vi "FPGA cRIOMain_v10.vi"() -> ()   [LabVIEW 2019]
doc: "Main FPGA VI\nUse the bitfile generated by this VI in the real-time code.\n\nv5: Use 16-pt MA filter in AI loop"
uses:
  TypeDefs/AO mode TabCtrl.ctl
  TypeDefs/SamplingModeEnum.ctl
  TypeDefs/AI_channelEnum.ctl
  <vilib>/Platform/TimedLoop/XDataNode/timing_clust.ctl
  <vilib>/Platform/TimedLoop/XDataNode/nitl_modes.ctl
  <vilib>/Platform/TimedLoop/XDataNode/wakeup.ctl
  <vilib>/rvi/Emulation/niFpgaGetClockAttributes.vi
  <vilib>/rvi/Emulation/niFpgaSctlEmulationGetInTimedLoop.vi
  <vilib>/rvi/Emulation/niFpgaEmulationReportErrorSimple.vi
  <vilib>/rvi/eio/common/nirviEmuTemplateMethod_errors.vi
  <vilib>/rvi/Emulation/niFpgaEmulationIsFPGAContextNoSignature.vi
  <vilib>/rvi/errors/niFpgaSetErrorForExecOnDevCompSimple.vi
  <vilib>/rvi/eio/common/nirviEmuReportErrorAndStop.vi
  <vilib>/rvi/DataTransferAndStorage/Container/Common/niFpgaContainerGetUniqueNameForEmu.vi
  <vilib>/rvi/FIFO/Fifo_Resource/nirvififoEmulationSetSize.vi
  <vilib>/rvi/FIFO/Fifo_Resource/nirviFifoEmulationQueueMgr.vi
  <instcachedir>/0/nirviFifoEmulationQueueMgr_E5CAEC123FF24DC58D834DCA3CDAA9B5.lvgen/nirviFifoEmulationQueueMgr_E5CAEC123FF24DC58D834DCA3CDAA9B5_000.vi
  <vilib>/rvi/FIFO/Fifo_Resource/nirvififoEmulationDetermineInputValidOut.vi
  <vilib>/rvi/FIFO/Fifo_Resource/nirvififoEmulationCreateLock.vi
  <vilib>/rvi/Emulation/niFpgaProcessEmulError.vi
  <vilib>/rvi/FIFO/Fifo_Resource/nirvififoEmulationObtainLock.vi
  <vilib>/rvi/FIFO/Fifo_Resource/nirvififoEmulationReleaseLock.vi
  <vilib>/rvi/occurrence/nirviWaitOnOccurrenceBase.vi
  <vilib>/rvi/errors/nirviReportUnexpectedCaseInternalError.vi
  <vilib>/rvi/errors/nirviReportUnexpectedCaseInternalError (U32).vi
  <vilib>/rvi/Emulation/niFpgaCriticalErrorInLSC.vi
  <instcachedir>/0/nirviFifoEmulationQueueMgr_E5CAEC123FF24DC58D834DCA3CDAA9B5.lvgen/nirviFifoEmulationQueueMgr_E5CAEC123FF24DC58D834DCA3CDAA9B5_006.vi
  <vilib>/Utility/error.llb/Clear Errors.vi
  <vilib>/rvi/Memory/Memory_Emulation/niFpgaMemoryEmulationCacheClearOnFirstRun.vi
  <vilib>/rvi/Memory/Memory_Emulation/nirvimemoryEmulationManagerCache_MakeExclusive.vi
  <vilib>/rvi/Memory/Memory_Emulation/niFpgaMemoryEmulationValidateCache.vi
  <vilib>/rvi/Memory/Memory_Emulation/nirvimemoryEmulationManagerCache_InsertValue.vi
  <vilib>/rvi/Memory/Memory_Emulation/nirvimemoryEmulationManagerCache_ReleaseExclusive.vi
  <vilib>/rvi/Memory/Memory_Emulation/nirvimemoryEmulationManagerCache_GetValue.vi
  <vilib>/rvi/Memory/Memory_Emulation/nirvimemoryEmulationManagerCache_SetValue.vi
  <vilib>/rvi/Analysis/common/codeGenErrors/XNode/niFpgaXNodeCodeGenErrorHandle.vi
  <vilib>/eio/EIONode/EIONode.xnode
  <vilib>/rvi/DataTransferAndStorage/Container/XNode/niFpgaContainer.xnode
  <vilib>/rvi/FIFO/Fifo_Resource/nirvififoEmulationWrite.vi
  <vilib>/rvi/FIFO/Fifo_Resource/nirvififoEmulationRead.vi
  <vilib>/rvi/DataTransferAndStorage/Register/Emulation/niFpgaRegisterEmulation.vi
  <vilib>/rvi/FXPMathLib/FxpMul/XNode/nifxpmath_Multiplier.xnode
  <vilib>/rvi/Analysis/measure/LMRsmpl/XNode/niFPGA Rational Resampler.xnode
  <vilib>/Platform/TimedLoop/XDataNode/XDataNode.xnode
  <vilib>/rvi/FXPMathLib/sim/FxpSim.dll
  <vilib>/Platform/TimedLoop/XDataNode/XDNodeRunTimeDep.lvlib
panel:
  out "AI M loop time [ticks]":u32
  out "FPGA AI DMA\nOverflow?":bool
  out "AI Processing\nLoop Rate to high?":bool
  in  "AI Process Time [ticks]":u32=125
  in  "Select Channel":T1
  out "Unable to\nsample at desired\nSample Rate?":bool
  out "Processing Loop time [ticks]":u32
  in  "Sampling Mode":T2
  in  "AO mode":T3
  in  "AO Out [V]":fxp<+/-,18,5> format="%#.6g"
  in  "AO enable?":bool
  out "AI In [V]":fxp<+/-,25,5> format="%#.6g"
  out "FPGA AO DMA\nOverflow?":bool
  out "Int. Output":fxp<+/-,20,5> format="%.17g"
  out "Raw AI Input":fxp<+/-,25,5> format="%.21g"
  in  "Sample Time [ticks]":u32=125
  out "AO Loop time [ticks]":u32
  out "AI Loop time [ticks]":u32
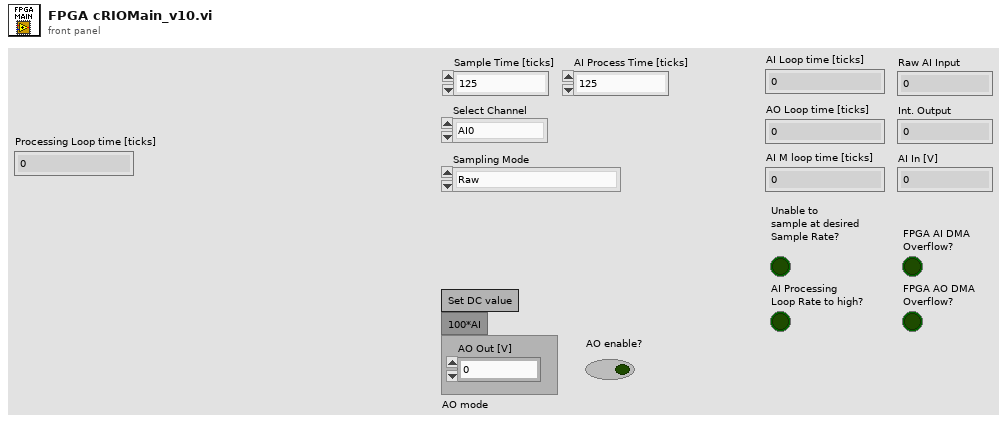
[diagram p1: front panel]
types:
  T1 = typedef "AI_channelEnum.ctl" = enum16{"AI0", "AI1", "AI2", "AI3"}
  T2 = typedef "SamplingModeEnum.ctl" = enum16{"Raw", "M64 (ReSpl)", "M128 (ReSpl)", "4pt MA (AI) + M64 (ReSpl)", "LPF (Proc.)", "4pt MA (AI) + LPF (Proc.)", "4pt MA (Proc.) + LPF (Proc.)"}
  T3 = typedef "AO mode TabCtrl.ctl" = enum32{"Set DC value", "100*AI"}
  T4 = typedef "XDNodeRunTimeDep.lvlib/timing_clust.ctl" = cluster{"Expected End [f-1]":u64, "Actual End [f-1]":u64, "Finished Late? [f-1]":bool, "Expected End [i-1]":u64, "Actual End [i-1]":u64, "Finished Late? [i-1]":bool, "Expected Start [i]":u64, "Actual Start [i]":u64, "Expected Start [f]":u64, "Actual Start [f]":u64, "Source Name":string, "Structure Name":string, "Period":i64, "Deadline":i64, "Offset":i64, "Start":i64, "Priority":i32, "Timeout":i32, "Mode":T5, "Wakeup Reason":T6, "Error":errorcluster, "Source Type":string, "Secondary Source Type":string, "Global End Time":u64, "Global Start Time":u64, "Frame Duration":u64, "Iteration Duration":u64, "Assigned CPU":i32, "I/O Scan Engine Mode":u32}
  T5 = typedef "XDNodeRunTimeDep.lvlib/nitl_modes.ctl" = enum32{"No Change", "Process missed periods, maintain original phase", "Discard missed periods, maintain original phase", "Process missed periods, ignore original phase", "Discard missed periods, ignore original phase"}
  T6 = typedef "XDNodeRunTimeDep.lvlib/wakeup.ctl" = enum32{"Normal", "Aborted", "Asynchronous wakeup", "Timing source error", "Timed loop error", "Timeout"}
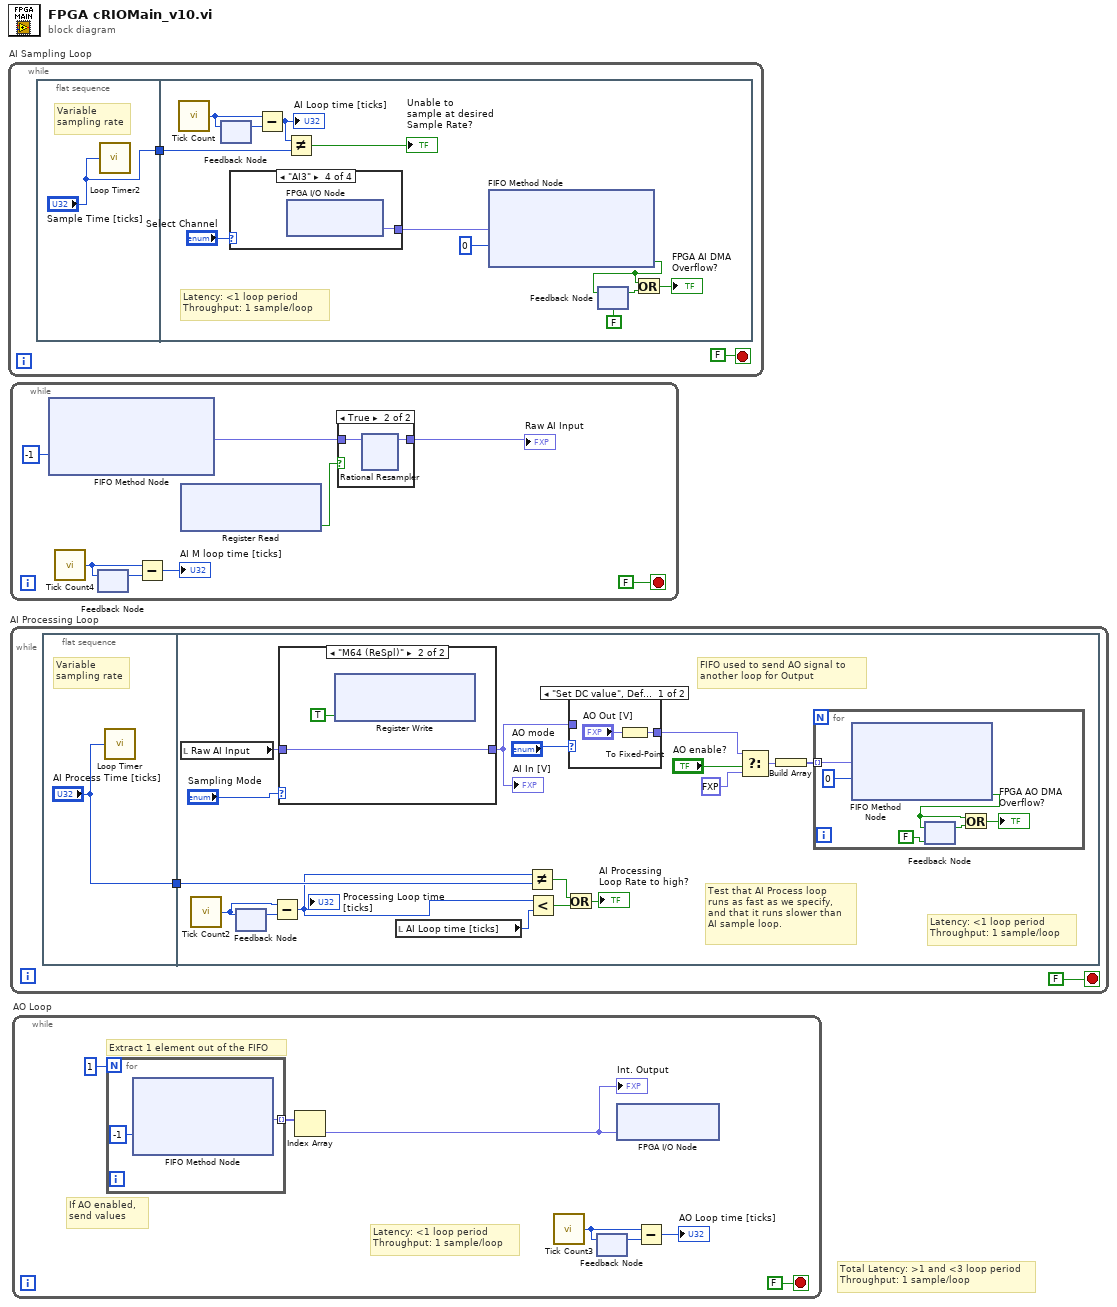
[diagram p0: block diagram]
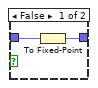
[diagram p2: hidden frame]
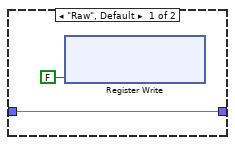
[diagram p3: hidden frame]
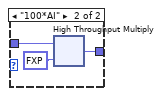
[diagram p4: hidden frame]
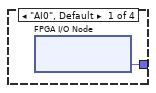
[diagram p5: hidden frame]
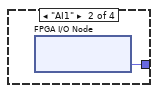
[diagram p6: hidden frame]
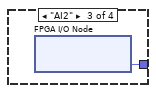
[diagram p7: hidden frame]
diagram:
  # "Total Latency: >1 and <3 loop period\nThroughput: 1 sample/loop"
  n1 = while "AI Sampling Loop" {
    stop <- FALSE stop-if-true
    n2 = flat-sequence {
      tunnel: ["Sample Time [ticks]"] -> w1
      tunnel: w1 -> [w12]
      frame #0 {
        # "Variable\nsampling rate"
        n3 = call "Loop Timer2"("Count(Ticks)"="Sample Time [ticks]") -> ()  [unwired: 1 out]
      }
      frame #1 {
        # "Latency: <1 loop period\nThroughput: 1 sample/loop"
        n4 = call "Tick Count"() -> ("Tick Count(Ticks)"=w15:u32)
        n5 = feedback #1() -> (w14:u32)  [unwired: 1 in]
        n6 = feedback-in #1(w15) -> ()
        n7 = case shown="\"AI3\"" "Select Channel" {
          tunnel: [w16 w17 w18 w19] -> w4
          frame "AI0", Default {
            n8 = xnode "FPGA I/O Node"() -> ("Mod4/AI0"=w16:fxp<+/-,24,5>)  [unwired: 1 in, 1 out]
          }
          frame "AI1" {
            n9 = xnode "FPGA I/O Node"() -> ("Mod4/AI1"=w17:fxp<+/-,24,5>)  [unwired: 1 in, 1 out]
          }
          frame "AI2" {
            n10 = xnode "FPGA I/O Node"() -> ("Mod4/AI2"=w18:fxp<+/-,24,5>)  [unwired: 1 in, 1 out]
          }
          frame "AI3" {
            n11 = xnode "FPGA I/O Node"() -> ("Mod4/AI3"=w19:fxp<+/-,24,5>)  [unwired: 1 in, 1 out]
          }
        }
        n12 = Subtract(x=w15, y=w14) -> (x-y=w13:u32)
        "AI Loop time [ticks]" <- w13
        n13 = Not Equal?(x=w13, y=w12) -> (x != y?=→"Unable to\nsample at desired\nSample Rate?":bool)
        n14 = xnode ("FIFO Method Node")("Element"=w4, "Timeout"=0) -> ("Timed Out?"=w7:bool)  [unwired: 1 in, 1 out]
        n15 = feedback #2(FALSE ("Timed Out?")) -> (w9:bool)
        n16 = feedback-in #2(w7) -> ()
        n17 = Or(x=w7, y=w9) -> (x .or. y?=→"FPGA AI DMA\nOverflow?":bool)
      }
    }
  }
  n18 = while {
    stop <- FALSE stop-if-true
    n19 = xnode ("FIFO Method Node")("Timeout"=-1) -> ("Element"=w21:fxp<+/-,24,5>)  [unwired: 1 in, 2 out]
    n20 = call "Tick Count4"() -> ("Tick Count(Ticks)"=w25:u32)
    n21 = feedback #3() -> (w24:u32)  [unwired: 1 in]
    n22 = feedback-in #3(w25) -> ()
    n23 = Subtract(x=w25, y=w24) -> (x-y=→"AI M loop time [ticks]":u32)
    n24 = xnode ("Register Read")() -> ("Data"=w22:bool)  [unwired: 1 in, 1 out]
    n25 = case shown="True" w22 {
      tunnel: w21 -> [w28 w31]
      tunnel: [w29 w30] -> w20
      frame False {
        n26 = To Fixed-Point(number=w28) -> (fixed-point=w29:fxp<+/-,25,5>)  [unwired: 1 in]
      }
      frame True {
        n27 = xnode "Rational Resampler"("input data"=w31) -> ("output data"=w30:fxp<+/-,25,5>)  [unwired: 2 out]
      }
    }
    "Raw AI Input" <- w20
  }
  n28 = while "AI Processing Loop" {
    stop <- FALSE stop-if-true
    n29 = flat-sequence {
      tunnel: ["AI Process Time [ticks]"] -> w66
      tunnel: w66 -> [w70]
      frame #0 {
        # "Variable\nsampling rate"
        n30 = call "Loop Timer"("Count(Ticks)"="AI Process Time [ticks]") -> ()  [unwired: 1 out]
      }
      frame #1 {
        # "Test that AI Process loop\nruns as fast as we specify,\nand that it runs slower than \nAI sample loop."
        # "Latency: <1 loop period\nThroughput: 1 sample/loop"
        # "FIFO used to send AO signal to \nanother loop for Output"
        n31 = local read "Raw AI Input"() -> (w74:fxp<+/-,25,5>)
        n32 = call "Tick Count2"() -> ("Tick Count(Ticks)"=w84:u32)
        n33 = feedback #4() -> (w85:u32)  [unwired: 1 in]
        n34 = feedback-in #4(w84) -> ()
        n35 = Subtract(x=w84, y=w85) -> (x-y=w69:u32)
        "Processing Loop time [ticks]" <- w69
        n36 = case shown="\"M64 (ReSpl)\"" "Sampling Mode" {
          tunnel: [w86 w88] -> w82
          tunnel: w74 -> [w86 w88]
          frame "Raw", Default {
            n37 = xnode ("Register Write")("Data"=FALSE) -> ()  [unwired: 1 in, 1 out]
          }
          frame "M64 (ReSpl)" {
            n38 = xnode ("Register Write")("Data"=TRUE) -> ()  [unwired: 1 in, 1 out]
          }
        }
        "AI In [V]" <- w82
        n39 = local read "AI Loop time [ticks]"() -> (w75:u32)
        n40 = Not Equal?(x=w69, y=w70) -> (x != y?=w72:bool)
        n41 = Less?(x=w69, y=w75) -> (x < y?=w71:bool)
        n42 = Or(x=w72, y=w71) -> (x .or. y?=→"AI Processing\nLoop Rate to high?":bool)
        n43 = case shown="\"Set DC value\", Default" "AO mode" {
          tunnel: [w91 w92] -> w79
          tunnel: w82 -> [_ w94]
          frame "Set DC value", Default {
            n44 = To Fixed-Point(number="AO Out [V]") -> (fixed-point=w91:fxp<+/-,20,5>)  [unwired: 1 in]
          }
          frame "100*AI" {
            n45 = xnode ("High Throughput Multiply")("x"=w94, "y"=fxp<+,5,7> 100.0) -> ("x*y"=w92:fxp<+/-,20,5>)
          }
        }
        n46 = Select(t=w79, s="AO enable?", f=fxp<+/-,20,5> 0.0) -> (s? t:f=w83:fxp<+/-,20,5>)
        n47 = Build Array(w83) -> (w78:fxp<+/-,20,5>[])
        n48 = for {
          tunnel: w78 -> [w95] mode=indexing
          n49 = xnode ("FIFO Method Node")("Element"=w95, "Timeout"=0) -> ("Timed Out?"=w96:bool)  [unwired: 1 in, 1 out]
          n50 = feedback-in #5(w96) -> ()
          n51 = feedback #5(FALSE ("Timed Out?")) -> (w99:bool)
          n52 = Or(x=w96, y=w99) -> (x .or. y?=→"FPGA AO DMA\nOverflow?":bool)
        }
      }
    }
  }
  n53 = while "AO Loop" {
    stop <- FALSE stop-if-true
    # "Latency: <1 loop period\nThroughput: 1 sample/loop"
    # "If AO enabled, \nsend values"
    # "Extract 1 element out of the FIFO"
    n54 = for {
      N: 1 -> [_]
      tunnel: [w109] -> w103 mode=indexing
      n55 = xnode ("FIFO Method Node")("Timeout"=-1) -> ("Element"=w109:fxp<+/-,20,5>)  [unwired: 1 in, 2 out]
    }
    n56 = Index Array(array=w103) -> (element=w101:fxp<+/-,20,5>)  [unwired: 1 in]
    "Int. Output" <- w101
    n57 = call "Tick Count3"() -> ("Tick Count(Ticks)"=w106:u32)
    n58 = feedback #6() -> (w105:u32)  [unwired: 1 in]
    n59 = feedback-in #6(w106) -> ()
    n60 = xnode "FPGA I/O Node"("Mod3/AO1"=w101) -> ()  [unwired: 1 in, 1 out]
    n61 = Subtract(x=w106, y=w105) -> (x-y=→"AO Loop time [ticks]":u32)
  }
